vi "Handle Error.vi"(8 "error in (no error)":errorcluster, 11 "CameraTestingUI in":refnum<class "CameraTestingENI.lvclass">) -> (0 "error out":errorcluster, 2 "stop actor?":bool=TRUE, 3 "CameraTestingUI out":refnum<class "CameraTestingENI.lvclass">)   [LabVIEW 2020, in "CameraTestingProxy.lvlib" / "CameraTestingENI.lvclass"]
doc: "(<B>Filename</B>: Actor Framework.lvlib:Actor.lvclass:Handle Error.vi)\n\nDefines how the actor handles an error that occurred while processing a message. By default, this method does nothing except stop the actor."
uses:
  CameraTestingENI.lvclass
  <vilib>/ActorFramework/Actor/Actor.lvclass
  CameraTestingENI.lvclass/CameraTestingENI.ctl
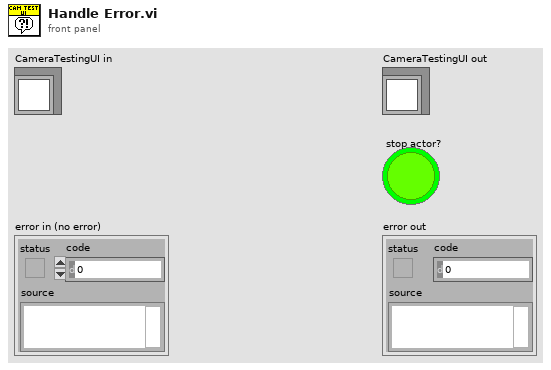
[diagram p1: front panel]
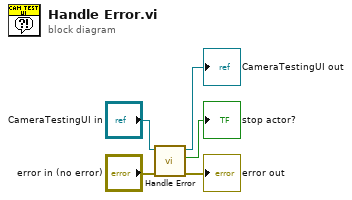
[diagram p0: block diagram]
diagram:
  n1 = call-parent "Handle Error.vi"("error in (no error)"="error in (no error)", "Actor in"="CameraTestingUI in") -> ("error out"=→"error out":errorcluster, "stop actor?"=→"stop actor?":bool, "Actor out"=→"CameraTestingUI out":refnum<class "CameraTestingENI.lvclass">)  [unwired: 7 in]
